vi "Ann_int.vi"(0 "Data":dbl[](array[numeric]), 1 "Loss Function":enum16{"MSE", "MAE"}(ring), 2 "Regularization":T1, 5 "Target":dbl format="%#_13g", 7 "Training?":bool, 9 "Parameters":T3, 13 "Adam Data In":T2) -> (4 "Output":dbl, 6 "Error":dbl, 10 "Adjusted Parameters":T3, 14 "Adam Data Out":T2)   [LabVIEW 2018]
uses:
  Sub-VI's/Adam_data.ctl
  Sub-VI's/Globals.vi
  Sub-VI's/Layer.vi
  Sub-VI's/Layer1d.vi
panel:
  out "Error Codes":i32[](array[numeric])
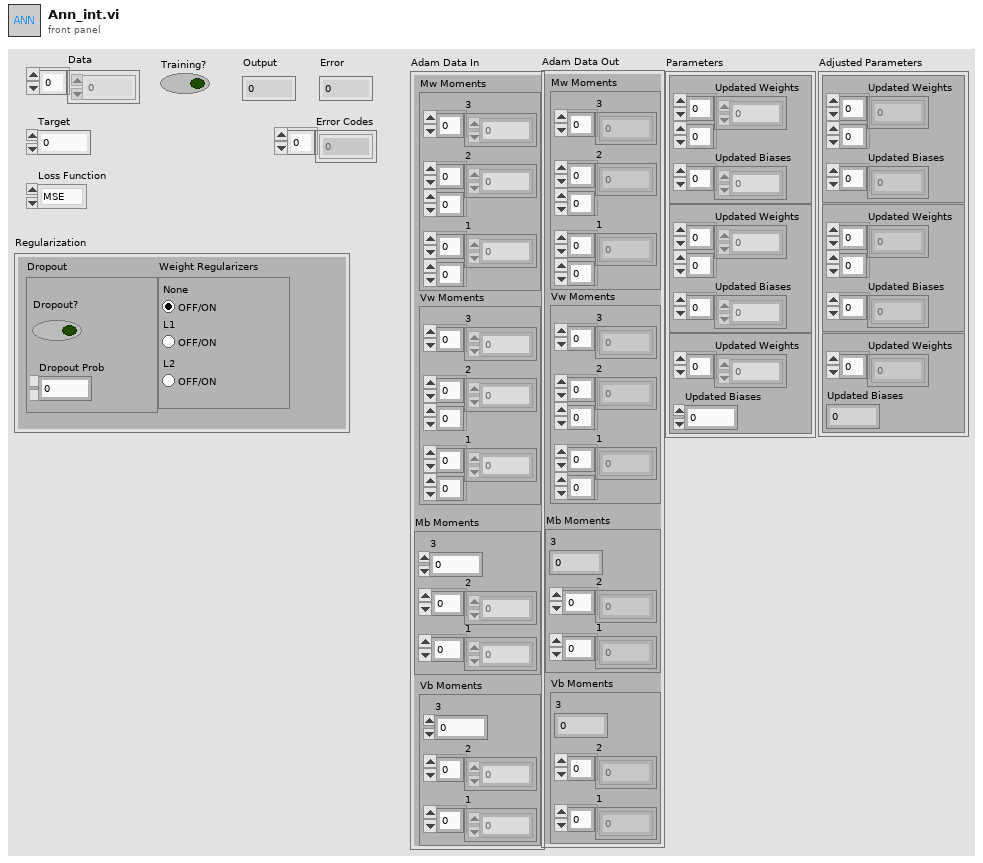
[diagram p1: front panel]
types:
  T1 = cluster{"Dropout":cluster{"Dropout?":bool, "Dropout Prob":dbl}, "Weight Regularizers":enum32{"None", "L1", "L2"}}
  T2 = typedef "Adam_data.ctl" = cluster{"Mw Moments":cluster{"3 ":dbl[], "2":dbl[][], "1":dbl[][]}, "Vw Moments":cluster{"3":dbl[], "2":dbl[][], "1":dbl[][]}, "Mb Moments":cluster{"3":dbl, "2":dbl[], "1":dbl[]}, "Vb Moments":cluster{"3":dbl, "2":dbl[], "1":dbl[]}}
  T3 = cluster{cluster{"Updated Weights":dbl[][], "Updated Biases":dbl[]}, cluster{"Updated Weights":dbl[][], "Updated Biases":dbl[]}, cluster{"Updated Weights":dbl[], "Updated Biases":dbl}}
  T4 = cluster{"Updated Weights":dbl[][], "Updated Biases":dbl[]}
  T5 = cluster{"Updated Weights":dbl[], "Updated Biases":dbl}
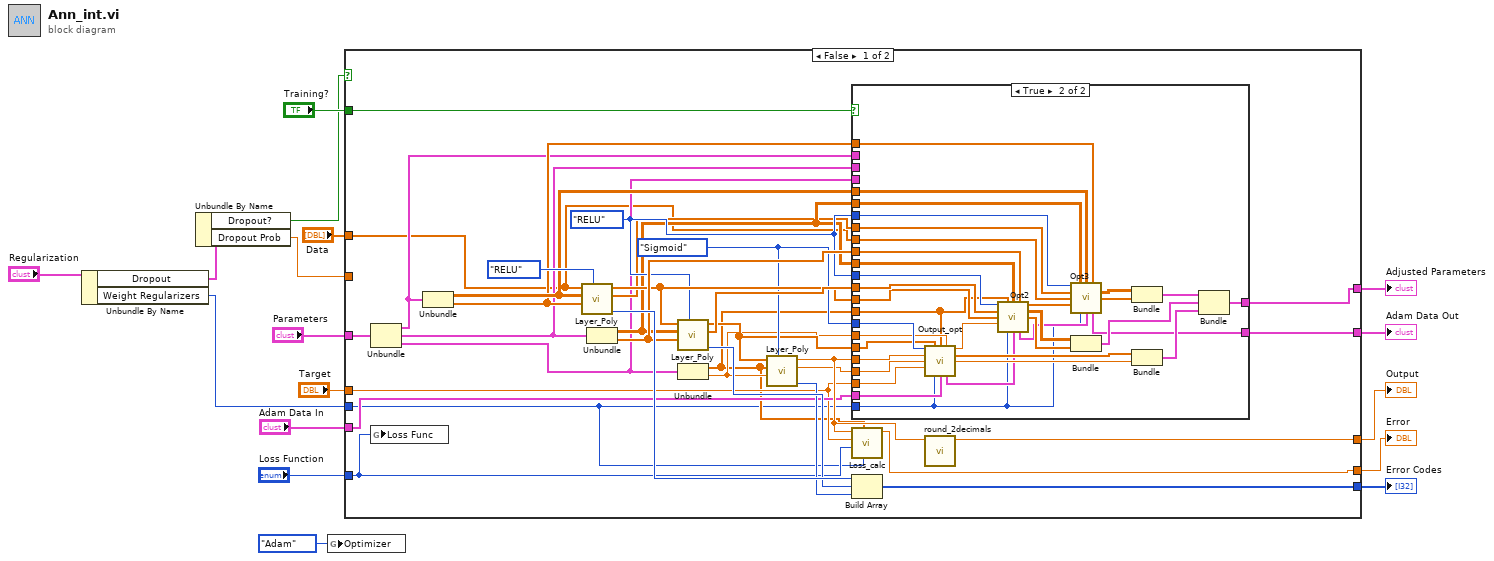
[diagram p0: block diagram]
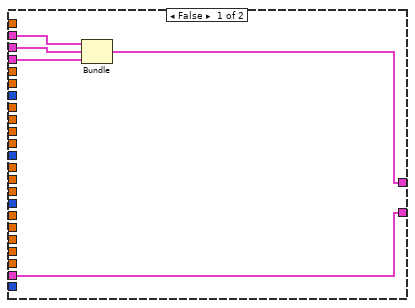
[diagram p2: hidden frame]
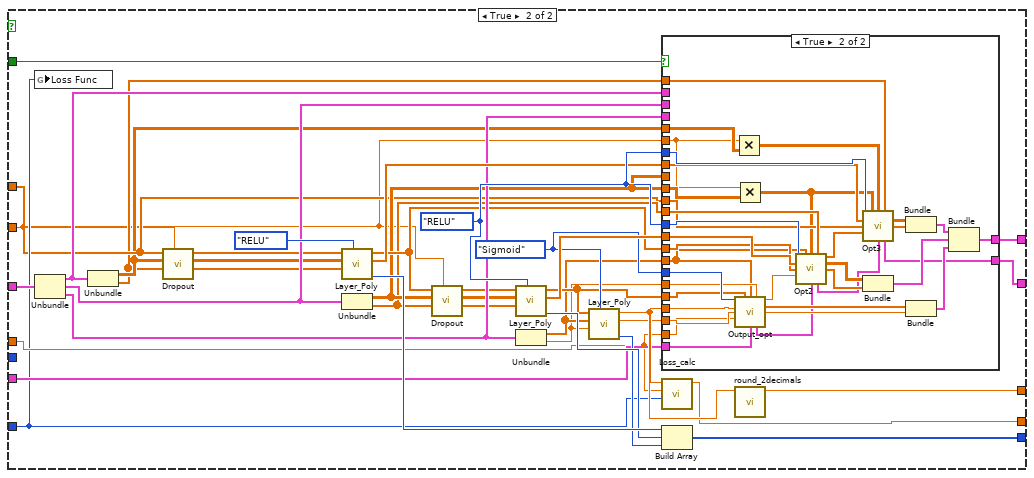
[diagram p3: hidden frame]
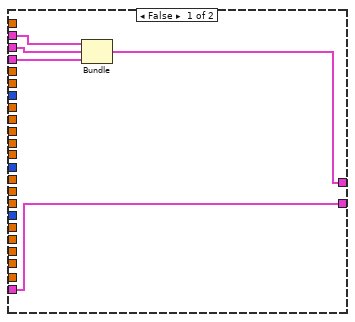
[diagram p4: hidden frame]
diagram:
  n1 = Unbundle By Name("Regularization") -> ("Dropout"=w4:cluster{"Dropout?":bool, "Dropout Prob":dbl}, "Weight Regularizers"=w1:enum32{"None", "L1", "L2"})
  n2 = Unbundle By Name(w4) -> ("Dropout?"=w3:bool, "Dropout Prob"=w2:dbl)
  n3 = global write "Globals.vi" "Optimizer"(enum16{"Adagrad", "Adadelta", "Adam"}."Adam" ("Optimizer")) -> ()
  n4 = case shown="False" w3 {
    tunnel: "Parameters" -> [w30 w113]
    tunnel: "Data" -> [w29 w97]
    tunnel: "Training?" -> [w28 w112]
    tunnel: "Adam Data In" -> [w27 w111]
    tunnel: [w26 w110] -> w12
    tunnel: [w25 w109] -> w11
    tunnel: "Target" -> [w24 w108]
    tunnel: [w23 w107] -> w9
    tunnel: [w22 w106] -> w8
    tunnel: "Loss Function" -> [w21 w105]
    tunnel: [w20 w104] -> w6
    tunnel: w2 -> [_ w91]
    tunnel: w1 -> [w18 _]
    frame False {
      w38 = enum32{"Sigmoid", "RELU", "Tanh", "Leaky RELU"}."Sigmoid" ("Activation Function")
      w43 = enum32{"Sigmoid", "RELU", "Tanh", "Leaky RELU"}."RELU" ("Activation Function")
      n5 = Unbundle(w30) -> (w34:T4, w33:T4, w32:T5)
      n6 = global write "Globals.vi" "Loss Func"(w21) -> ()
      n7 = Unbundle(w34) -> ("Updated Weights"=w41:dbl[][], "Updated Biases"=w40:dbl[])
      n8 = call-poly "Layer_Poly.vi"("Activation Function"=enum32{"Sigmoid", "RELU", "Tanh", "Leaky RELU"}."RELU", "Biases"=w40, "Weights"=w41, "Data"=w29) -> ("Error"=w50:i32, "Net Activation"=w39:dbl[], "Output"=w44:dbl[])  [unwired: 5 in]
      n9 = Unbundle(w33) -> ("Updated Weights"=w42:dbl[][], "Updated Biases"=w46:dbl[])
      n10 = call-poly "Layer_Poly.vi"("Activation Function"=w43, "Biases"=w46, "Weights"=w42, "Data"=w44) -> ("Error"=w49:i32, "Net Activation"=w45:dbl[], "Output"=w37:dbl[])  [unwired: 5 in]
      n11 = Unbundle(w32) -> ("Updated Weights"=w19:dbl[], "Updated Biases"=w31:dbl)
      n12 = call-poly "Layer_Poly.vi"("Activation Function"=w38, "Biases"=w31, "Weights"=w19, "Data"=w37) -> ("Error"=w48:i32, "Net Activation"=w35:dbl, "Output"=w36:dbl)  [unwired: 5 in]
      n13 = case shown="True" w28 {
        tunnel: w43 -> [_ w90]
        tunnel: w42 -> [_ w89]
        tunnel: w46 -> [_ w88]
        tunnel: w45 -> [_ w87]
        tunnel: w44 -> [_ w86]
        tunnel: w43 -> [_ w85]
        tunnel: w42 -> [_ w84]
        tunnel: w41 -> [_ w83]
        tunnel: w40 -> [_ w82]
        tunnel: w39 -> [_ w81]
        tunnel: w29 -> [_ w80]
        tunnel: w38 -> [_ w78]
        tunnel: w37 -> [_ w77]
        tunnel: w36 -> [_ w76]
        tunnel: w35 -> [_ w75]
        tunnel: w24 -> [_ w74]
        tunnel: [w52 w59] -> w26
        tunnel: w34 -> [w55 _]
        tunnel: w33 -> [w54 _]
        tunnel: w32 -> [w53 _]
        tunnel: w19 -> [_ w66]
        tunnel: w31 -> [_ w67]
        tunnel: [w51 w58] -> w25
        tunnel: w27 -> [w51 w57]
        tunnel: w18 -> [_ w56]
        frame False {
          n14 = Bundle(w55, w54, w53) -> (w52:T3)  [unwired: 1 in]
        }
        frame True {
          n15 = call "Output_opt.vi"("Activation Function"=w78, "Activation l-1"=w77, "Weights"=w66, "Biases"=w67, "Activation"=w76, "Net Output"=w75, "Target"=w74, "Weight Regularizers"=w56, "Adam Data In"=w57) -> ("Delta"=w73:dbl, "Updated Weights"=w70:dbl[], "Updated Biases"=w69:dbl, "Adam Data Out"=w61:T2)  [unwired: 3 in]
          n16 = call "Opt2.vi"("Activation Function"=w90, "Weights l+1"=w66, "Weights"=w89, "Biases"=w88, "Net Output"=w87, "Activations l-1"=w86, "Delta l+1"=w73, "Weight Regularizers"=w56, "Adam Data In"=w61) -> ("Delta l"=w79:dbl[], "Updated Weights"=w65:dbl[][], "Updated Biases"=w64:dbl[], "Adam Data Out"=w60:T2)  [unwired: 3 in]
          n17 = call "Opt3.vi"("Activation Function"=w85, "Weights l+1"=w84, "Weights"=w83, "Biases"=w82, "Net Output"=w81, "Activations l-1"=w80, "Delta l+1"=w79, "Weight Regularizers"=w56, "Adam Data In"=w60) -> ("Updated Weights"=w63:dbl[][], "Updated Biases"=w62:dbl[], "Adam Data Out"=w58:T2)  [unwired: 4 in]
          n18 = Bundle("Updated Weights"=w65, "Updated Biases"=w64) -> (w72:T4)  [unwired: 1 in]
          n19 = Bundle("Updated Weights"=w63, "Updated Biases"=w62) -> (w71:T4)  [unwired: 1 in]
          n20 = Bundle("Updated Weights"=w70, "Updated Biases"=w69) -> (w68:T5)  [unwired: 1 in]
          n21 = Bundle(w71, w72, w68) -> (w59:T3)  [unwired: 1 in]
        }
      }
      n22 = call "Loss_calc.vi"("Weight Regularizers"=w18, "Weights"=w19, "Loss Type"=w21, "Target"=w24, "Data"=w36) -> ("Loss"=w23:dbl)  [unwired: 6 in]
      n23 = Build Array(w50, w49, w48) -> (w22:i32[])
      n24 = call "round_2decimals.vi"("Number"=w36) -> ("Rounded Number"=w20:dbl)  [unwired: 10 in]
    }
    frame True {
      w122 = enum32{"Sigmoid", "RELU", "Tanh", "Leaky RELU"}."Sigmoid" ("Activation Function")
      w124 = enum32{"Sigmoid", "RELU", "Tanh", "Leaky RELU"}."RELU" ("Activation Function")
      n25 = global write "Globals.vi" "Loss Func"(w105) -> ()
      n26 = Unbundle(w113) -> (w118:T4, w117:T4, w116:T5)
      n27 = Unbundle(w118) -> ("Updated Weights"=w96:dbl[][], "Updated Biases"=w95:dbl[])
      n28 = call "Dropout.vi"("Droput Prob"=w91, "Biases"=w95, "Weights"=w96, "Data"=w97) -> ("Droupout Biases"=w92:dbl[], "Dropout Weights"=w93:dbl[][], "Droput Data"=w94:dbl[])  [unwired: 5 in]
      n29 = call-poly "Layer_Poly.vi"("Activation Function"=enum32{"Sigmoid", "RELU", "Tanh", "Leaky RELU"}."RELU", "Biases"=w92, "Weights"=w93, "Data"=w94) -> ("Error"=w129:i32, "Net Activation"=w123:dbl[], "Output"=w103:dbl[])  [unwired: 5 in]
      n30 = Unbundle(w117) -> ("Updated Weights"=w102:dbl[][], "Updated Biases"=w101:dbl[])
      n31 = call "Dropout.vi"("Droput Prob"=w91, "Biases"=w101, "Weights"=w102, "Data"=w103) -> ("Droupout Biases"=w98:dbl[], "Dropout Weights"=w99:dbl[][], "Droput Data"=w100:dbl[])  [unwired: 5 in]
      n32 = call-poly "Layer_Poly.vi"("Activation Function"=w124, "Biases"=w98, "Weights"=w99, "Data"=w100) -> ("Error"=w128:i32, "Net Activation"=w125:dbl[], "Output"=w121:dbl[])  [unwired: 5 in]
      n33 = Unbundle(w116) -> ("Updated Weights"=w115:dbl[], "Updated Biases"=w114:dbl)
      n34 = call-poly "Layer_Poly.vi"("Activation Function"=w122, "Biases"=w114, "Weights"=w115, "Data"=w121) -> ("Error"=w127:i32, "Net Activation"=w119:dbl, "Output"=w120:dbl)  [unwired: 5 in]
      n35 = case shown="True" w112 {
        tunnel: w124 -> [_ w170]
        tunnel: w102 -> [_ w139]
        tunnel: w101 -> [_ w169]
        tunnel: w125 -> [_ w168]
        tunnel: w103 -> [_ w167]
        tunnel: w124 -> [_ w166]
        tunnel: w102 -> [_ _]
        tunnel: w96 -> [_ w137]
        tunnel: w95 -> [_ w165]
        tunnel: w123 -> [_ w164]
        tunnel: w97 -> [_ w163]
        tunnel: w122 -> [_ w161]
        tunnel: w121 -> [_ w160]
        tunnel: w120 -> [_ w159]
        tunnel: w119 -> [_ w158]
        tunnel: w108 -> [_ w157]
        tunnel: [w131 w142] -> w110
        tunnel: w118 -> [w134 _]
        tunnel: w117 -> [w133 _]
        tunnel: w116 -> [w132 _]
        tunnel: w115 -> [_ w149]
        tunnel: w114 -> [_ w150]
        tunnel: [w130 w141] -> w109
        tunnel: w111 -> [w130 w140]
        tunnel: w91 -> [_ w135]
        frame False {
          n36 = Bundle(w134, w133, w132) -> (w131:T3)  [unwired: 1 in]
        }
        frame True {
          n37 = Multiply(x=w135, y=w137) -> (x*y=w136:dbl[][])
          n38 = Multiply(x=w135, y=w139) -> (x*y=w138:dbl[][])
          n39 = call "Output_opt.vi"("Activation Function"=w161, "Activation l-1"=w160, "Weights"=w149, "Biases"=w150, "Activation"=w159, "Net Output"=w158, "Target"=w157, "Adam Data In"=w140) -> ("Delta"=w156:dbl, "Updated Weights"=w153:dbl[], "Updated Biases"=w152:dbl, "Adam Data Out"=w144:T2)  [unwired: 4 in]
          n40 = call "Opt2.vi"("Activation Function"=w170, "Weights l+1"=w149, "Weights"=w138, "Biases"=w169, "Net Output"=w168, "Activations l-1"=w167, "Delta l+1"=w156, "Adam Data In"=w144) -> ("Delta l"=w162:dbl[], "Updated Weights"=w148:dbl[][], "Updated Biases"=w147:dbl[], "Adam Data Out"=w143:T2)  [unwired: 4 in]
          n41 = call "Opt3.vi"("Activation Function"=w166, "Weights l+1"=w138, "Weights"=w136, "Biases"=w165, "Net Output"=w164, "Activations l-1"=w163, "Delta l+1"=w162, "Adam Data In"=w143) -> ("Updated Weights"=w146:dbl[][], "Updated Biases"=w145:dbl[], "Adam Data Out"=w141:T2)  [unwired: 5 in]
          n42 = Bundle("Updated Weights"=w148, "Updated Biases"=w147) -> (w155:T4)  [unwired: 1 in]
          n43 = Bundle("Updated Weights"=w146, "Updated Biases"=w145) -> (w154:T4)  [unwired: 1 in]
          n44 = Bundle("Updated Weights"=w153, "Updated Biases"=w152) -> (w151:T5)  [unwired: 1 in]
          n45 = Bundle(w154, w155, w151) -> (w142:T3)  [unwired: 1 in]
        }
      }
      n46 = call "Loss_calc.vi"("Loss Type"=w105, "Target"=w108, "Data"=w120) -> ("Loss"=w107:dbl)  [unwired: 8 in]
      n47 = Build Array(w129, w128, w127) -> (w106:i32[])
      n48 = call "round_2decimals.vi"("Number"=w120) -> ("Rounded Number"=w104:dbl)  [unwired: 10 in]
    }
  }
  "Adjusted Parameters" <- w12
  "Adam Data Out" <- w11
  "Error" <- w9
  "Error Codes" <- w8
  "Output" <- w6
